vi "Function.vi"(8 "error in (no error)":errorcluster, 10 "Value":timestamp, 11 "Two Terminal in":refnum<class "Increment_Time.lvclass">) -> (0 "error out":errorcluster, 2 "Result":timestamp, 3 "Two Terminal out":refnum<class "Increment_Time.lvclass">)   [LabVIEW 2021, in "Increment_Time.lvclass"]
uses:
  Increment_Time.lvclass
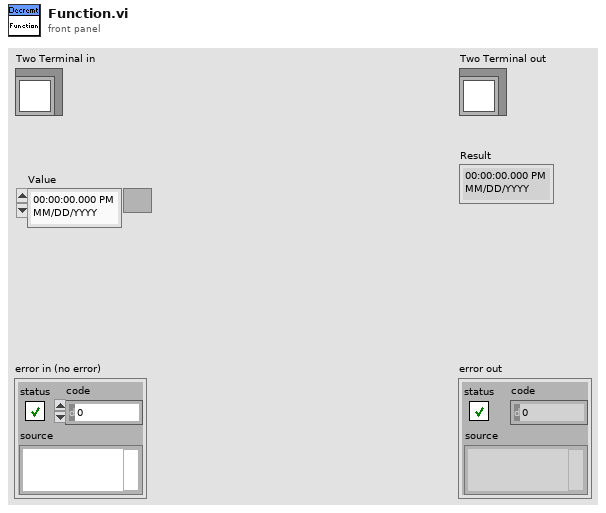
[diagram p1: front panel]
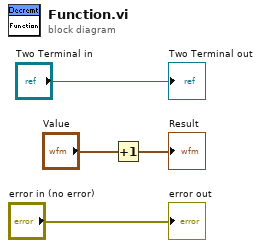
[diagram p0: block diagram]
diagram:
  n1 = Increment(x="Value") -> (x+1=→"Result":timestamp)
  "error out" <- "error in (no error)"
  "Two Terminal out" <- "Two Terminal in"
